vi "Pre Launch Init.vi"(11 "Console in":refnum<class "Console.lvclass">) -> (0 "error out":errorcluster, 3 "Console out":refnum<class "Console.lvclass">)   [LabVIEW 2015, in "EditPanel API.lvlib" / "Console.lvclass"]
doc: "(<B>Filename</B>: Actor Framework.lvlib:Actor.lvclass:Pre Launch Init.vi)\n\nDefines behavior that occurs after the Launch Nested Actor method is invoked but before the actor's Actor Core method begins running.\n\nBy default, this method does nothing. A descendant class may override it to define behavior."
uses:
  Console.lvclass
  Type Definition/Console_Q Data Type.ctl
  Console Reply/Console Reply/Console Reply.lvclass
  Panel Control_Interface/Panel_interface/Panel Controller Interface.lvclass
  <vilib>/ActorFramework/Actor/Actor.lvclass/Actor.ctl
  <vilib>/ActorFramework/Message Enqueuer/Message Enqueuer.lvclass/Message Enqueuer.ctl
  Console.lvclass/Console.ctl
  Console Reply/Console Reply/Console Reply.lvclass/Console Reply.ctl
  <vilib>/ActorFramework/Message Enqueuer/Init from Existing Queue.vi
  <vilib>/ActorFramework/Message Enqueuer/Enqueue.vi
  <vilib>/ActorFramework/Message Priority Queue/Priority Enqueue.vi
  <vilib>/ActorFramework/Message Enqueuer/Message Enqueuer.lvclass
  Panel Request/Panel Request Launch Console/Panel Request Launch Console.lvclass
  <vilib>/ActorFramework/Actor/Actor.lvclass
  EditPanel_class/EditPanel API.lvclass
  <vilib>/ErrorRing/Error Ring.xnode
  <vilib>/Utility/error.llb/Error Cluster From Error Code.vi
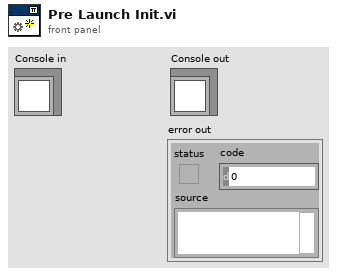
[diagram p1: front panel]
types:
  T1 = typedef "EditPanel API.lvlib/Console.lvclass/Console_Q Data Type.ctl" = cluster{"Console Reply":refnum<class "Console Reply.lvclass">, "Panel":refnum<class "Panel Controller Interface.lvclass">}
  T2 = enum16{"Attach", "Detach", "Flush", "Update", "Get"}
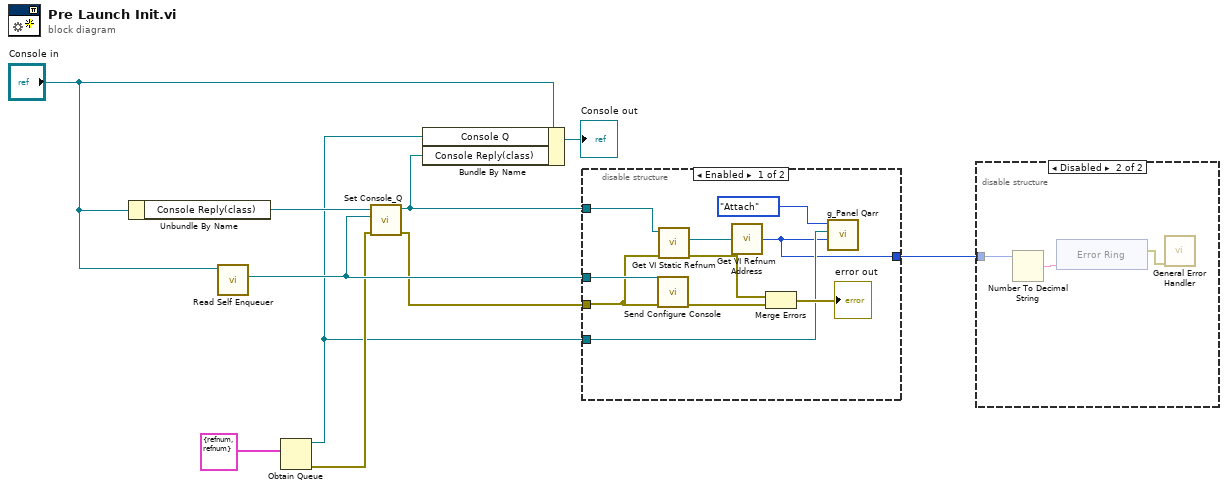
[diagram p0: block diagram]
diagram:
  n1 = Unbundle By Name("Console in") -> ("Console Reply(class)"=w7:refnum<class "Console Reply.lvclass">)
  n2 = call <vilib>:"Read Self Enqueuer.vi"("Actor"="Console in") -> ("Self Enqueuer"=w6:refnum<class "Message Enqueuer.lvclass">)  [unwired: 10 in]
  n3 = Obtain Queue(element data type=T1 {"Console Reply"=refnum, "Panel"=refnum}) -> (queue out=w2:refnum<queue>, error out=w5:errorcluster)  [unwired: 4 in, 1 out]
  n4 = call "Set Console_Q.vi"("error in (no error)"=w5, "Console Q"=w6, "Console Reply.lvclass"=w7) -> ("error out"=w4:errorcluster, "Console Reply.lvclass out"=w3:refnum<class "Console Reply.lvclass">)  [unwired: 7 in]
  n5 = Bundle By Name(cluster="Console in", "Console Q"=w2, "Console Reply(class)"=w3) -> (→"Console out":refnum<class "Console.lvclass">)
  n6 = disable-structure shown="Enabled" {
    disable-tunnel: w6 -> [w20 _]
    disable-tunnel: w4 -> [w16 _]
    disable-tunnel: w3 -> [w13 _]
    disable-tunnel: w2 -> [w12 _]
    disable-tunnel: [w11 _] -> w1
    frame Enabled {
      n7 = call "Send Configure Console.vi"("error in (no error)"=w16, "Message Enqueuer"=w20) -> ("error out"=w18:errorcluster)  [unwired: 8 in, 1 out]
      n8 = call "Get VI Static Refnum.vi"("error in (no error)"=w16, "Console Reply in"=w13) -> ("error out"=w14:errorcluster, "VI Static Refnum"=w15:refnum<vi>)  [unwired: 7 in, 1 out]
      n9 = call "Get VI Refnum Address.vi"("VI Refnum"=w15) -> ("Get Ref Address"=w11:u16)
      n10 = Merge Errors(w14, w18) -> (→"error out":errorcluster)
      n11 = call "g_Panel Qarr.vi"("VI Address"=w11, "Console Q"=w12, "Operation"=T2."Attach") -> ()  [unwired: 8 in, 1 out]
    }
    frame Disabled {
    }
  }
  n12 = disable-structure shown="Disabled" {
    disable-tunnel: w1 -> [_ w23]
    frame Enabled {
    }
    frame Disabled {
      n13 = Number To Decimal String(number=w23) -> (decimal integer string=w22:string)  [unwired: 1 in]
      n14 = xnode "Error Ring"("parameter 0"=w22) -> ("error out"=w21:errorcluster)
      n15 = call <vilib>:"General Error Handler.vi"("error in (no error)"=w21) -> ()  [unwired: 10 in, 5 out]
    }
  }
